vi "execute-exe.vi"(8 "error in (no error)":errorcluster caption="错误输入（无错误）") -> (0 "error out":errorcluster caption="错误输出", 11 "添加的路径":path)   [LabVIEW 2013]
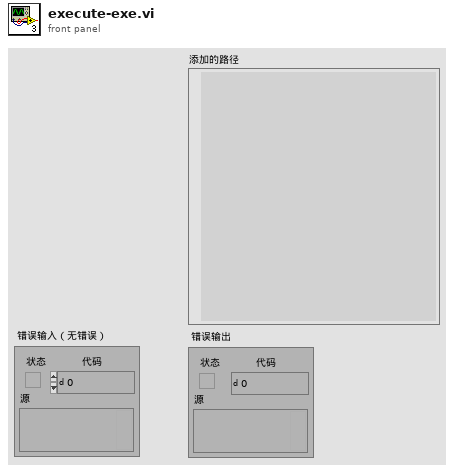
[diagram p1: front panel]
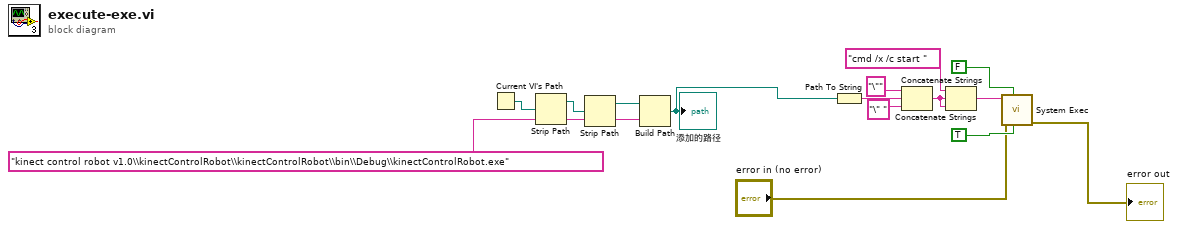
[diagram p0: block diagram]
diagram:
  n1 = Current VI's Path() -> (path=w7:path)
  n2 = Strip Path(path=w7) -> (stripped path=w6:path)  [unwired: 1 out]
  n3 = Strip Path(path=w6) -> (stripped path=w5:path)  [unwired: 1 out]
  n4 = Build Path(base path=w5, name or relative path="kinect control robot v1.0\\kinectControlRobot\\kinectControlRobot\\bin\\Debug\\kinectControlRobot.exe" ("名称或相对路径")) -> (appended path=w3:path)
  "添加的路径" <- w3
  n5 = Path To String(path=w3) -> (string=w12:string)
  n6 = Concatenate Strings("\"" ("Substring"), w12, "\" " ("Substring")) -> (w13:string)
  n7 = Concatenate Strings("cmd /x /c start ", w13, w13) -> (w9:string)
  n8 = call <vilib>:"System Exec.vi"("run minimized? (F)"=TRUE, "wait until completion? (T)"=FALSE ("Wait until done"), "error in (no error)"="error in (no error)", "command line"=w9) -> ("error out"=→"error out":errorcluster)  [unwired: 2 in, 5 out]
